vi "AgPSA _Reset.vi"(8 "error in (no error)":errorcluster, 11 "PSA In":refnum<visa-resource-name>) -> (0 "error out":errorcluster, 3 "PSA Out":refnum<visa-resource-name>)   [LabVIEW 2015]
uses:
  <instrlib>/Agilent ESA PSA Series/Agilent ESA PSA Series.lvlib
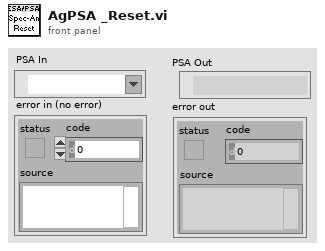
[diagram p1: front panel]
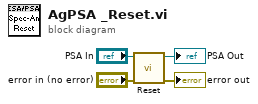
[diagram p0: block diagram]
diagram:
  n1 = call <instrlib>:"Reset.vi"("error in (no error)"="error in (no error)", "VISA resource name"="PSA In") -> ("error out"=→"error out":errorcluster, "VISA resource name out"=→"PSA Out":refnum<visa-resource-name>)  [unwired: 8 in]
